vi "Create.vi"(7 "Virtual Mode":T1, 8 "error in":errorcluster, 9 "HOME?":bool, 10 "Project Path":path, 11 "Init Mode":T2) -> (0 "error out":errorcluster, 3 "Gantry out":refnum<class "Gantry.lvclass">)   [LabVIEW 2026, in "Gantry.lvclass"]
uses:
  Gantry.lvclass
  Type Definitions/Init_Modes.ctl
  Type Definitions/Virtual Modes.ctl
  Gantry.lvclass/Gantry.ctl
  GH2/GH2.lvclass
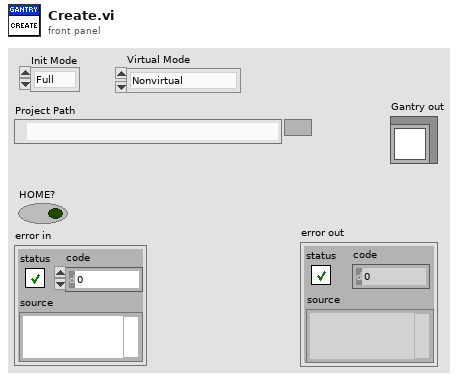
[diagram p1: front panel]
types:
  T1 = typedef "Virtual Modes.ctl" = enum16{"Nonvirtual", "Virtual"}
  T2 = typedef "Init_Modes.ctl" = enum16{"Full", "Robot Only", "Dispenser Only", "Cameras Only", "Robot and Cameras", "Robot and Cameras and Dispenser", "Manifold Only"}
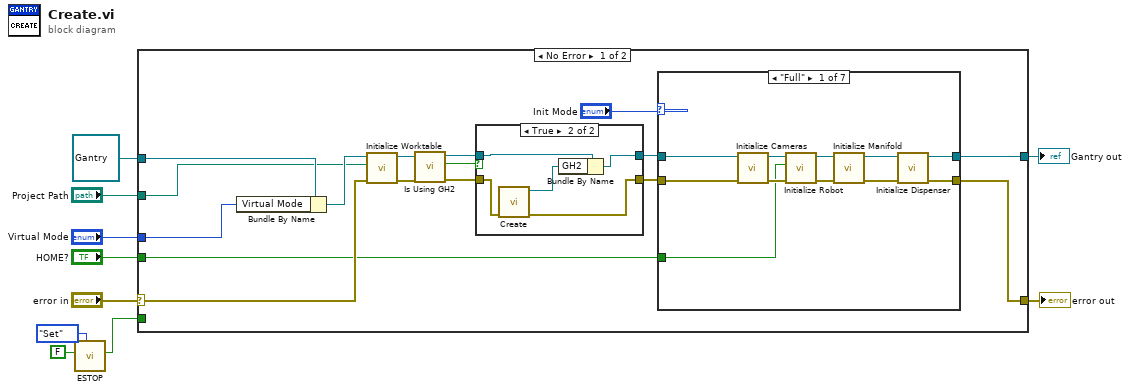
[diagram p0: block diagram]
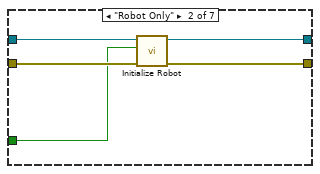
[diagram p3: hidden frame]
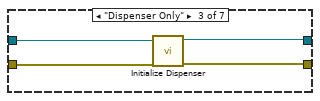
[diagram p4: hidden frame]
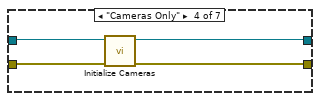
[diagram p5: hidden frame]
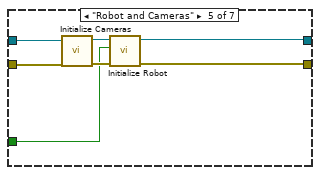
[diagram p6: hidden frame]
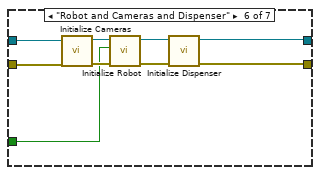
[diagram p7: hidden frame]
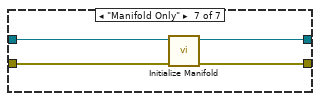
[diagram p8: hidden frame]
diagram:
  n1 = call "ESTOP.vi"("Get/Set"=enum16{"Get", "Set"}."Set", "Value In"=FALSE) -> ("Value Out"=w3:bool)  [unwired: 9 in]
  n2 = case shown="No Error" "error in" {
    selector: "error in" -> [w23 w79]
    tunnel: [w25 w79] -> w9
    tunnel: [w26 w78] -> w7
    tunnel: refnum<class "Gantry.lvclass"> refnum ("Gantry Class in") -> [w24 w78]
    tunnel: "Project Path" -> [w19 _]
    tunnel: w3 -> [_ _]
    tunnel: "Virtual Mode" -> [w20 _]
    tunnel: "HOME?" -> [w18 _]
    frame No Error {
      n3 = Bundle By Name(cluster=w24, "Virtual Mode"=w20) -> (w22:refnum<class "Gantry.lvclass">)
      n4 = call-dynamic "Initialize Worktable.vi"("error in"=w23, "Project Path"=w19, "Gantry in"=w22) -> ("error out"=w16:errorcluster, "Gantry out"=w17:refnum<class "Gantry.lvclass">)  [unwired: 7 in]
      n5 = call "Is Using GH2.vi"("error in (no error)"=w16, "Gantry in"=w17) -> ("error out"=w13:errorcluster, "Using GH2"=w15:bool, "Gantry out"=w14:refnum<class "Gantry.lvclass">)  [unwired: 7 in]
      n6 = case shown="True" w15 {
        tunnel: w14 -> [w28 w32]
        tunnel: w13 -> [w27 w33]
        tunnel: [w28 w30] -> w12
        tunnel: [w27 w29] -> w11
        frame False {
        }
        frame True {
          n7 = call "Create.vi"("error in (no error)"=w33) -> ("error out"=w29:errorcluster, "GH2 out"=w31:refnum<class "GH2.lvclass">)  [unwired: 9 in]
          n8 = Bundle By Name(cluster=w32, "GH2"=w31) -> (w30:refnum<class "Gantry.lvclass">)
        }
      }
      n9 = case shown="\"Full\"" "Init Mode" {
        tunnel: [w44 w47 w50 w55 w60 w66 w77] -> w26
        tunnel: [w43 w46 w51 w54 w59 w65 w76] -> w25
        tunnel: w12 -> [w40 w49 w53 w57 w62 w71 w75]
        tunnel: w11 -> [w37 w48 w52 w56 w61 w70 w74]
        tunnel: w18 -> [w34 w45 _ _ w58 w69 _]
        frame "Full" {
          n10 = call-dynamic "Initialize Cameras.vi"("error in"=w37, "Gantry in"=w40) -> ("error out"=w36:errorcluster, "Gantry out"=w39:refnum<class "Gantry.lvclass">)  [unwired: 8 in]
          n11 = call-dynamic "Initialize Robot.vi"("error in"=w36, "HOME?"=w34, "Gantry in"=w39) -> ("error out"=w35:errorcluster, "Gantry out"=w38:refnum<class "Gantry.lvclass">)  [unwired: 7 in]
          n12 = call-dynamic "Initialize Manifold.vi"("error in"=w35, "Gantry in"=w38) -> ("error out"=w41:errorcluster, "Gantry out"=w42:refnum<class "Gantry.lvclass">)  [unwired: 8 in]
          n13 = call-dynamic "Initialize Dispenser.vi"("error in"=w41, "Gantry in"=w42) -> ("error out"=w43:errorcluster, "Gantry out"=w44:refnum<class "Gantry.lvclass">)  [unwired: 8 in]
        }
        frame "Robot Only" {
          n14 = call-dynamic "Initialize Robot.vi"("error in"=w48, "HOME?"=w45, "Gantry in"=w49) -> ("error out"=w46:errorcluster, "Gantry out"=w47:refnum<class "Gantry.lvclass">)  [unwired: 7 in]
        }
        frame "Dispenser Only" {
          n15 = call-dynamic "Initialize Dispenser.vi"("error in"=w52, "Gantry in"=w53) -> ("error out"=w51:errorcluster, "Gantry out"=w50:refnum<class "Gantry.lvclass">)  [unwired: 8 in]
        }
        frame "Cameras Only" {
          n16 = call-dynamic "Initialize Cameras.vi"("error in"=w56, "Gantry in"=w57) -> ("error out"=w54:errorcluster, "Gantry out"=w55:refnum<class "Gantry.lvclass">)  [unwired: 8 in]
        }
        frame "Robot and Cameras" {
          n17 = call-dynamic "Initialize Cameras.vi"("error in"=w61, "Gantry in"=w62) -> ("error out"=w63:errorcluster, "Gantry out"=w64:refnum<class "Gantry.lvclass">)  [unwired: 8 in]
          n18 = call-dynamic "Initialize Robot.vi"("error in"=w63, "HOME?"=w58, "Gantry in"=w64) -> ("error out"=w59:errorcluster, "Gantry out"=w60:refnum<class "Gantry.lvclass">)  [unwired: 7 in]
        }
        frame "Robot and Cameras and Dispenser" {
          n19 = call-dynamic "Initialize Cameras.vi"("error in"=w70, "Gantry in"=w71) -> ("error out"=w72:errorcluster, "Gantry out"=w73:refnum<class "Gantry.lvclass">)  [unwired: 8 in]
          n20 = call-dynamic "Initialize Robot.vi"("error in"=w72, "HOME?"=w69, "Gantry in"=w73) -> ("error out"=w67:errorcluster, "Gantry out"=w68:refnum<class "Gantry.lvclass">)  [unwired: 7 in]
          n21 = call-dynamic "Initialize Dispenser.vi"("error in"=w67, "Gantry in"=w68) -> ("error out"=w65:errorcluster, "Gantry out"=w66:refnum<class "Gantry.lvclass">)  [unwired: 8 in]
        }
        frame "Manifold Only" {
          n22 = call-dynamic "Initialize Manifold.vi"("error in"=w74, "Gantry in"=w75) -> ("error out"=w76:errorcluster, "Gantry out"=w77:refnum<class "Gantry.lvclass">)  [unwired: 8 in]
        }
      }
    }
    frame Error {
    }
  }
  "error out" <- w9
  "Gantry out" <- w7
